vi "Write False by Value.vi"(8 "Error In":errorcluster, 11 "Writer In":refnum<class "Writer.lvclass">) -> (0 "Error Out":errorcluster, 3 "Writer Out":refnum<class "Writer.lvclass">)   [LabVIEW 2017, in "LabPack.lvlib" / "Writer.lvclass"]
uses:
  Writer.lvclass
  Writer.lvclass/Writer.ctl
  Public/Status/Read Is Error.vi
  Public/Status/Read Status.vi
  Public/Status/Read Status Message.vi
  Utility/Status Code.vi
  <vilib>/Utility/error.llb/Error Cluster From Error Code.vi
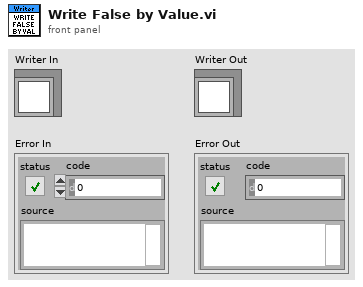
[diagram p1: front panel]
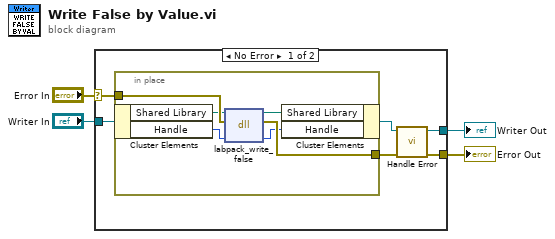
[diagram p0: block diagram]
diagram:
  n1 = case shown="No Error" "Error In" {
    selector: "Error In" -> [w10 w18]
    tunnel: [w5 w18] -> w3
    tunnel: "Writer In" -> [w9 w17]
    tunnel: [w7 w17] -> w1
    frame No Error {
      n2 = in-place {
        in-place-border: w10 -> [w16]
        in-place-border: [w15] -> w6
        n3 = in-place-cluster #1(w9) -> ("Shared Library"=w14:path, "Handle"=w12:u64)
        n4 = dll-call lib="D:/Users/cfield/Code/MessagePack/LabPack/LabVIEW/trunk/src/LabPack/Private/labpack-x64.dll" fn="labpack_write_false"(path in=w14, error in=w16, "writer"=w12) -> (path out=w13:path, error out=w15:errorcluster, "writer"=w11:u64)  [unwired: 2 in]
        n5 = in-place-cluster #1("Shared Library"=w13, "Handle"=w11) -> (w8:refnum<class "Writer.lvclass">)
      }
      n6 = call "Handle Error.vi"("Error In"=w6, "Writer In"=w8) -> ("Error Out"=w5:errorcluster, "Writer Out"=w7:refnum<class "Writer.lvclass">)  [unwired: 8 in]
    }
    frame Error {
    }
  }
  "Error Out" <- w3
  "Writer Out" <- w1
